vi "Post-Project-Copying Process.vi"(10 "MetaDataObj":refnum<class "MetaDataObj.lvclass">) -> ()   [LabVIEW 2021, in "Plugin Generator.lvlib"]
uses:
  Plugin Generator.lvlib
  PluginGenerator_MetaDataObj/PluginGenerator_MetaDataObj.lvclass
  SubVIs/[Global].vi
  ed511516-c131-45ea-930f-d7c7c2eb0895.vi
  <resource>/dialog/NewProjectWizard/MetaDataObj/MetaDataObj.lvclass
panel:
  out "Progress":string
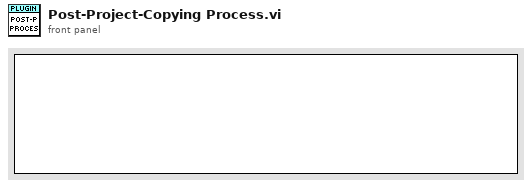
[diagram p1: front panel]
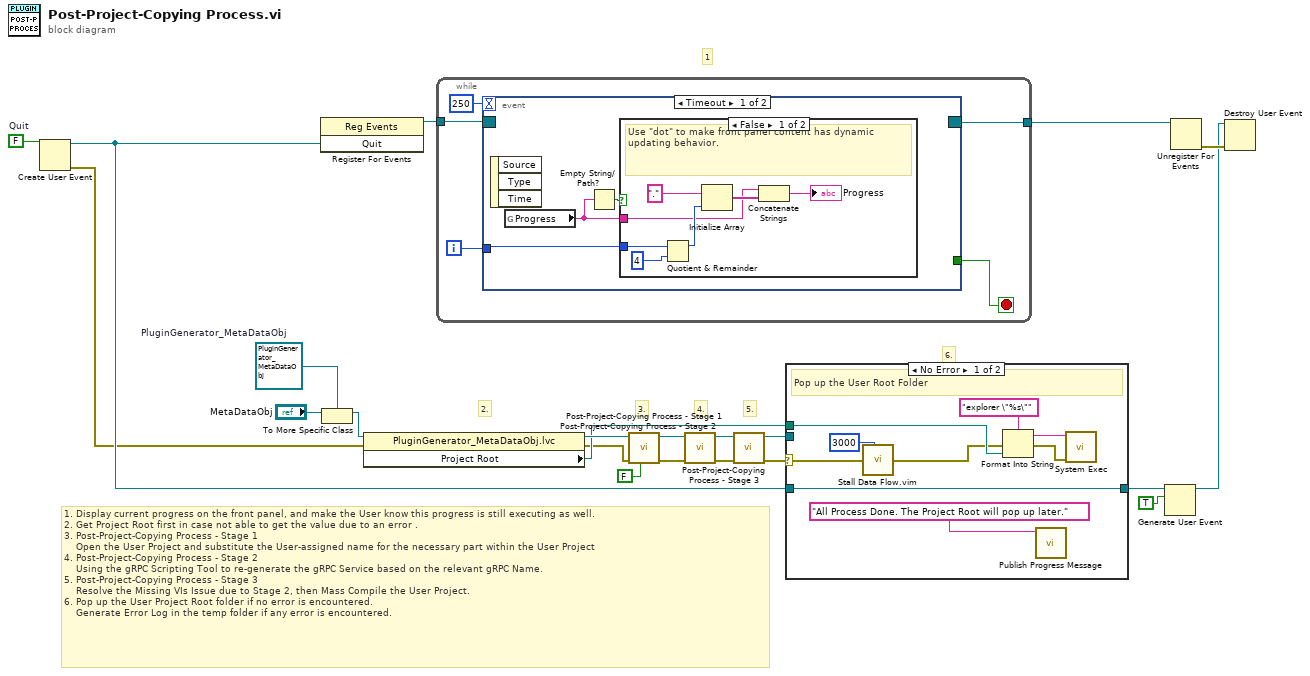
[diagram p0: block diagram]
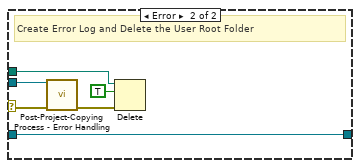
[diagram p2: hidden frame]
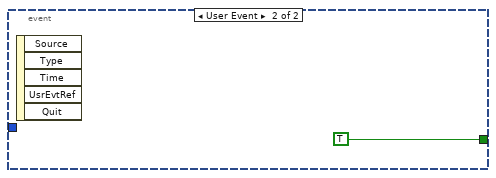
[diagram p4: hidden frame]
diagram:
  w15 = FALSE  # Quit
  w21 = refnum<class "PluginGenerator_MetaDataObj.lvclass"> refnum  # PluginGenerator_MetaDataObj
  # "6."
  # "5."
  # "4."
  # "3."
  # "1. Display current progress on the front panel, and make the User know this progress is still executing as well.\n2. Get Project Root first in case not able to get the value due to an error .\n3. Post-Project-Copying Process - Stage 1\n    Open the User Project and substitute the User-assigned name for the necessary part within the User Project\n4. Post-Project-Copying Process - Stage 2\n    Using the gRPC Scripting Tool to re-generate the gRPC Service based on the relevant gRPC Name.\n5. Post-Project-Copying Process - Stage 3\n    Resolve the Missing VIs Issue due to Stage 2, then Mass Compile the User Project.\n6. Pop up the User Project Root folder if no error is encountered.\n    Generate Error Log in the temp folder if any error is encountered."
  # "2."
  # "1"
  n1 = Create User Event(user event datatype=w15) -> (user event=w8:refnum<user-event>, error out=w5:errorcluster)  [unwired: 1 in]
  n2 = register-events(w8) -> (reference out=w14:refnum<event-registration>)  [unwired: 2 in, 1 out]
  n3 = To More Specific Class(target class=w21, reference="MetaDataObj") -> (specific class reference=w7:refnum<class "PluginGenerator_MetaDataObj.lvclass">)  [unwired: 1 in, 1 out]
  n4 = property class="PluginGenerator_MetaDataObj.lvc"(reference=w7, error in=w5) -> (reference out=w6:refnum<class "PluginGenerator_MetaDataObj.lvclass">, error out=w1:errorcluster, "Project Root"=w3:path)
  n5 = while {
    tunnel: w14 -> [w26]
    tunnel: [w23] -> w12
    i -> [w24]
    stop <- w25 stop-if-true
    n6 = event shown="[0] Timeout" {
      selector: w26 -> [_ _]
      dyn-events: [_ _] -> w23
      timeout: 250 -> [_ _]
      tunnel: [_ TRUE] -> w25
      tunnel: w24 -> [w28 _]
      event Timeout {
        n7 = event-data() -> ()  [unwired: 1 in, 3 out]
        n8 = global read "[Global].vi" "Progress"() -> (w29:string)
        n9 = Empty String/Path?(string/path=w29) -> (empty?=w30:bool)
        n10 = case shown="False" w30 {
          tunnel: w29 -> [w34 _]
          tunnel: w28 -> [w32 _]
          frame False {
            # "Use \"dot\" to make front panel content has dynamic updating behavior."
            n11 = Quotient & Remainder(x=w32, y=4) -> (x-y*floor(x/y)=w37:i32)  [unwired: 1 out]
            n12 = Initialize Array(".", w37) -> (w35:string[])
            n13 = Concatenate Strings(w34, w35) -> (→"Progress":string)
          }
          frame True {
            # "No dynamic update front panel content due to progress not starting yet."
          }
        }
      }
      event User Event {
        n14 = event-data() -> ()  [unwired: 1 in, 5 out]
      }
    }
  }
  n15 = call "Post-Project-Copying Process - Stage 1.vi"("Debug"=FALSE, "error in"=w1, "PluginGenerator_MetaDataObj"=w6) -> ("error out"=w18:errorcluster, "PluginGenerator_MetaDataObj out"=w17:refnum<class "PluginGenerator_MetaDataObj.lvclass">)  [unwired: 6 in, 1 out]
  n16 = call "Post-Project-Copying Process - Stage 2.vi"("error in"=w18, "PluginGenerator_MetaDataObj"=w17) -> ("error out"=w20:errorcluster, "PluginGenerator_MetaDataObj out"=w16:refnum<class "PluginGenerator_MetaDataObj.lvclass">)  [unwired: 8 in]
  n17 = call "Post-Project-Copying Process - Stage 3.vi"("error in"=w20, "PluginGenerator_MetaDataObj"=w16) -> ("error out"=w4:errorcluster, "PluginGenerator_MetaDataObj out"=w2:refnum<class "PluginGenerator_MetaDataObj.lvclass">)  [unwired: 8 in]
  n18 = case shown="No Error" w4 {
    selector: w4 -> [w41 w52]
    tunnel: [w44 w53] -> w9
    tunnel: w8 -> [w44 w53]
    tunnel: w3 -> [w43 w49]
    tunnel: w2 -> [_ w51]
    frame No Error {
      # "Pop up the User Root Folder"
      n19 = call "Stall Data Flow.vim"("value in"=w41, "milliseconds to wait"=u32 3000) -> ("value out"=w40:errorcluster)  [unwired: 1 out]
      n20 = Format Into String(format string="explorer \"%s\"", error in=w40, w43) -> (resulting string=w47:string, error out=w45:errorcluster)  [unwired: 1 in]
      n21 = call "Publish Progress Message.vi"("Progress"="All Process Done. The Project Root will pop up later.") -> ()  [unwired: 11 in]
      n22 = call <vilib>:"System Exec.vi"("error in (no error)"=w45, "command line"=w47) -> ()  [unwired: 6 in, 4 out]
    }
    frame Error {
      # "Create Error Log and Delete the User Root Folder"
      n23 = call "Post-Project-Copying Process - Error Handling.vi"("error in"=w52, "PluginGenerator_MetaDataObj"=w51) -> ("error out"=w50:errorcluster)  [unwired: 8 in, 1 out]
      n24 = Delete(path (use dialog)=w49, entire hierarchy (F)=TRUE, error in=w50) -> ()  [unwired: 2 in, 3 out]
    }
  }
  n25 = Generate User Event(user event=w9, event data cluster=TRUE ("event data")) -> (user event out=w10:refnum<user-event>)  [unwired: 2 in, 1 out]
  n26 = Unregister For Events(event registration refnum=w12) -> (error out=w11:errorcluster)  [unwired: 1 in]
  n27 = Destroy User Event(user event=w10, error in=w11) -> ()  [unwired: 1 out]
